vi "Kick_Main.vi"() -> ()   [LabVIEW 2017]
panel:
  out "Number of Matches Returned":i32
  out "Circles":T1(array[cluster]) {"Position"."Y" format="%.2f"; "Position"."X" format="%.2f"}
  in  "Threshold Value":sgl=1.0 format="%.2f"
  out "Vertical Edges":T2(array[cluster]) {"Point2 (Real-World)"."Y" format="%.2f"; "Point2 (Real-World)"."X" format="%.2f"; "Point1 (Real-World)"."Y" format="%.2f"; "Point1 (Real-World)"."X" format="%.2f"; "Point2 (Pixels)"."Y" format="%.2f"; "Point2 (Pixels)"."X" format="%.2f"; "Point1 (Pixels)"."Y" format="%.2f"; "Point1 (Pixels)"."X" format="%.2f"}
  out "Horizontal Edges":T2(array[cluster]) {"Point2 (Real-World)"."Y" format="%.2f"; "Point2 (Real-World)"."X" format="%.2f"; "Point1 (Real-World)"."Y" format="%.2f"; "Point1 (Real-World)"."X" format="%.2f"; "Point2 (Pixels)"."Y" format="%.2f"; "Point2 (Pixels)"."X" format="%.2f"; "Point1 (Pixels)"."Y" format="%.2f"; "Point1 (Pixels)"."X" format="%.2f"}
  out "error out 2":errorcluster
  out "error out":errorcluster
  out "Image":T3(plugin-control)
  in  "Calibration":path
  in  "Image":path
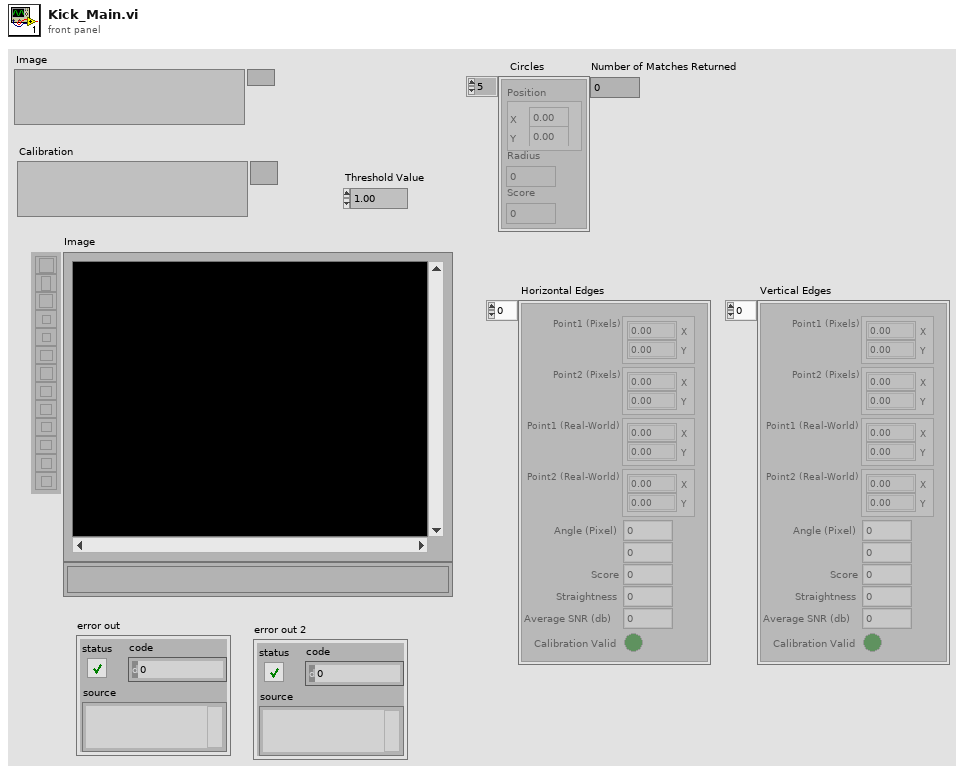
[diagram p1: front panel]
types:
  T1 = cluster{"Position":cluster{"X":sgl, "Y":sgl}, "Radius":dbl, "Score":dbl}[]
  T2 = cluster{"Point1 (Pixels)":cluster{"X":sgl, "Y":sgl}, "Point2 (Pixels)":cluster{"X":sgl, "Y":sgl}, "Point1 (Real-World)":cluster{"X":sgl, "Y":sgl}, "Point2 (Real-World)":cluster{"X":sgl, "Y":sgl}, "Angle (Pixel)":dbl, "Angle (Real-World)":dbl, "Score":dbl, "Straightness":dbl, "Average SNR (db)":dbl, "Calibration Valid":bool}[]
  T3 = typedef "IMAQ Image.ctl" = refnum<image>
  T4 = typedef "IMAQ Coordinate System" = cluster{"Reference System":cluster{"Origin":cluster{"X":sgl, "Y":sgl}, "Angle (deg)":sgl, "Axis Reference":u32}, "Measurement System":cluster{"Origin":cluster{"X":sgl, "Y":sgl}, "Angle (deg)":sgl, "Axis Reference":u32}}
  T5 = typedef "Image Unit" = enum32{"Undefined", "Angström", "Micrometer", "Millimeter", "Centimeter", "Meter", "Kilometer", "Microinch", "Inch", "Feet", "Nautical miles", "Standard miles", "Steps"}
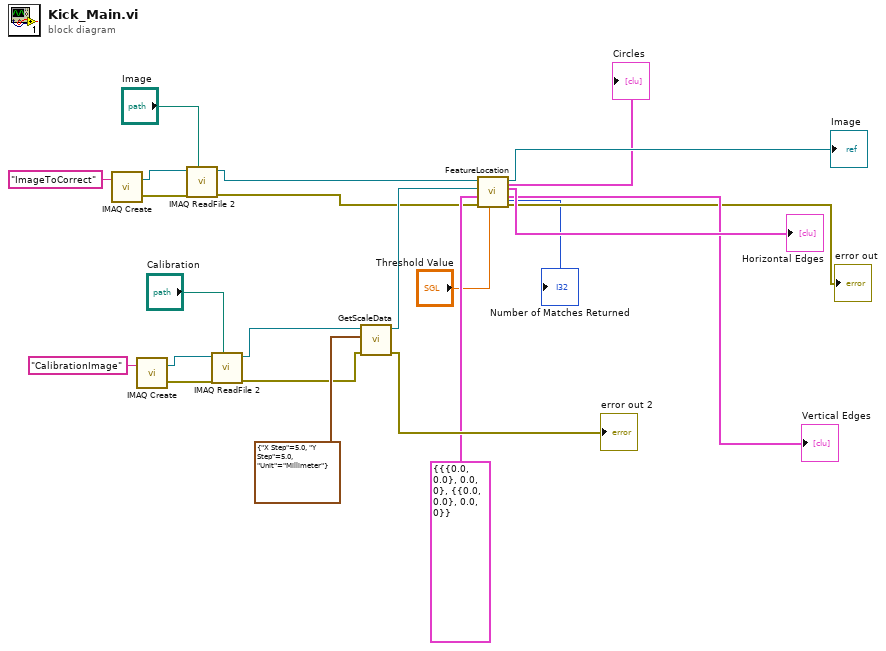
[diagram p0: block diagram]
diagram:
  n1 = call "IMAQ Create"("Image Name"="ImageToCorrect") -> ("New Image"=w22:T3, "error out"=w20:errorcluster)  [unwired: 4 in]
  n2 = call "IMAQ Create"("Image Name"="CalibrationImage") -> ("New Image"=w18:T3, "error out"=w16:errorcluster)  [unwired: 4 in]
  n3 = call "IMAQ ReadFile 2"("File Path"="Image", "error in (no error)"=w20, "Image"=w22) -> ("error out"=w8:errorcluster, "Image Out"=w11:T3)  [unwired: 4 in, 3 out]
  n4 = call "IMAQ ReadFile 2"("File Path"="Calibration", "error in (no error)"=w16, "Image"=w18) -> ("error out"=w13:errorcluster, "Image Out"=w15:T3)  [unwired: 4 in, 3 out]
  n5 = call "GetScaleData.vi"("error in (no error)"=w13, "Grid Descriptor"=cluster{"X Step":sgl, "Y Step":sgl, "Unit":T5} {"X Step"=5.0, "Y Step"=5.0, "Unit"=enum."Millimeter"}, "Image Src"=w15) -> ("error out"=→"error out 2":errorcluster, "Image"=w10:T3)  [unwired: 7 in]
  n6 = call "FeatureLocation.vi"("Threshold Value"="Threshold Value", "error in (no error)"=w8, "Coordinate System"=T4 {"Reference System"={"Origin"={"X"=0.0, "Y"=0.0}, "Angle (deg)"=0.0, "Axis Reference"=0}, "Measurement System"={"Origin"={"X"=0.0, "Y"=0.0}, "Angle (deg)"=0.0, "Axis Reference"=0}}, "Calibration Data"=w10, "Image"=w11) -> ("error out"=→"error out":errorcluster, "Vertical Edges"=→"Vertical Edges":T2, "Horizontal Edges"=→"Horizontal Edges":T2, "Image 2"=→"Image":T3, "Number of Matches Returned"=→"Number of Matches Returned":i32, "Circles"=→"Circles":T1)  [unwired: 1 in]
